vi "Initialize_Ocean_Optics_USB_2000_4000.vi"(6 "Enable Strobe (Disabled)":bool, 8 "VISA resource name":refnum<visa-resource-name>, 9 "Working Directory":string, 10 "End Wavelength (< 1040 nm)":dbl format="%#_13g", 11 "Start Wavelength (> 340 nm)":dbl format="%#_13g") -> (0 "Wavelength (nm)":dbl[](array[numeric]), 1 "error out":errorcluster, 2 "Length of Spec Data to Keep":dbl, 3 "Start Index of Spec Data to Keep":dbl, 4 "VISA resource name out":refnum<visa-resource-name>)   [LabVIEW 2012]
uses:
  <vilib>/Utility/file.llb/Write To Spreadsheet File (DBL).vi
  <instrlib>/Ocean Optics 2000 4000/Ocean Optics 2000 4000.lvlib
panel:
  in  "Spectrometer Wavelength Resolution (nm)":dbl=0.21328
  in  "Spectrometer Lowest Wavelength (nm)":dbl=340.488
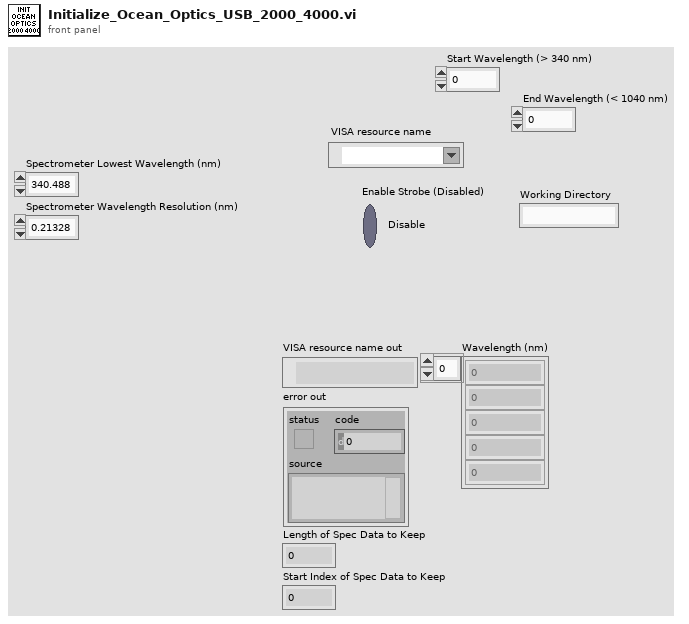
[diagram p1: front panel]
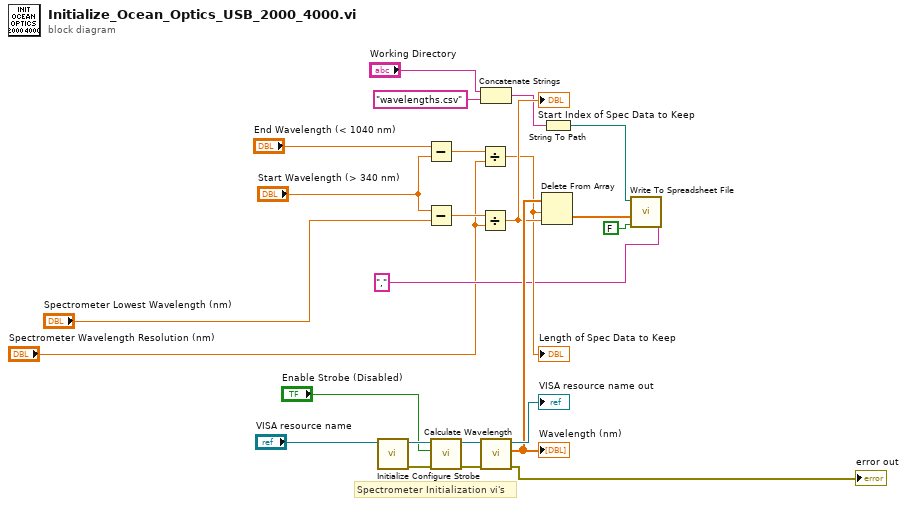
[diagram p0: block diagram]
diagram:
  # "Spectrometer Initialization vi's"
  n1 = call <instrlib>:"Initialize.vi"("VISA resource name"="VISA resource name") -> ("error out"=w23:errorcluster, "VISA resource name out"=w24:refnum<visa-resource-name>)  [unwired: 2 in, 7 out]
  n2 = Subtract(x="End Wavelength (< 1040 nm)", y="Start Wavelength (> 340 nm)") -> (x-y=w10:dbl)
  n3 = Subtract(x="Start Wavelength (> 340 nm)", y="Spectrometer Lowest Wavelength (nm)") -> (x-y=w14:dbl)
  n4 = call "Configure Strobe.vi"("error in (no error)"=w23, "Enable Strobe (Disabled)"="Enable Strobe (Disabled)", "VISA resource name"=w24) -> ("error out"=w17:errorcluster, "VISA resource name out"=w18:refnum<visa-resource-name>)  [unwired: 7 out]
  n5 = Divide(x=w10, y="Spectrometer Wavelength Resolution (nm)") -> (x/y=w9:dbl)
  "Length of Spec Data to Keep" <- w9
  n6 = Divide(x=w14, y="Spectrometer Wavelength Resolution (nm)") -> (x/y=w13:dbl)
  "Start Index of Spec Data to Keep" <- w13
  n7 = Concatenate Strings("Working Directory", "wavelengths.csv") -> (w5:string)
  n8 = call <instrlib>:"Calculate Wavelength.vi"("error in (no error)"=w17, "VISA resource name"=w18) -> ("error out"=→"error out":errorcluster, "Wavelength (nm)"=w16:dbl[], "VISA resource name out"=→"VISA resource name out":refnum<visa-resource-name>)  [unwired: 1 in, 6 out]
  "Wavelength (nm)" <- w16
  n9 = Delete From Array(array=w16, length=w9, index=w13) -> (deleted portion=w15:dbl[])  [unwired: 1 out]
  n10 = String To Path(string=w5) -> (path=w7:path)
  n11 = call-poly <vilib>:"Write To Spreadsheet File.vi"("delimiter (\\t)"=",", "append to file? (new file:F)"=FALSE, "1D data"=w15, "file path (dialog if empty)"=w7) -> ()  [unwired: 4 in, 1 out]
